vi "Get DDG External Output Time.vi"(8 "error in (no error)":errorcluster, 9 "puiWidth":cluster{}, 10 "puiDelay":cluster{}, 11 "uiIndex":u32) -> (0 "error out":errorcluster, 1 "puiWidth out":cluster{}, 2 "puiDelay out":cluster{}, 3 "function return":u32)   [LabVIEW 2014, in "atmcd32d.lvlib"]
doc: "unsigned int WINAPI GetDDGExternalOutputTime(at_u32 uiIndex, at_u64 * puiDelay, at_u64 * puiWidth);"
uses:
  atmcd32d.lvlib
  atmcd32d.dll
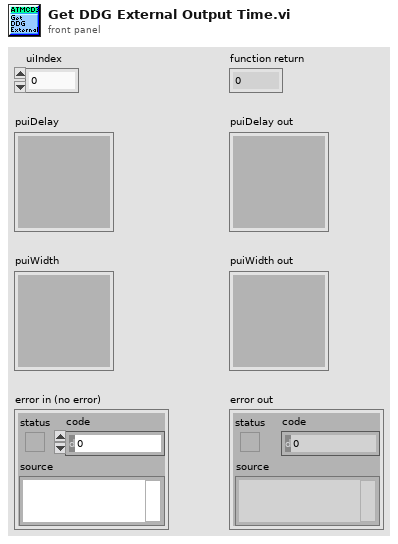
[diagram p1: front panel]
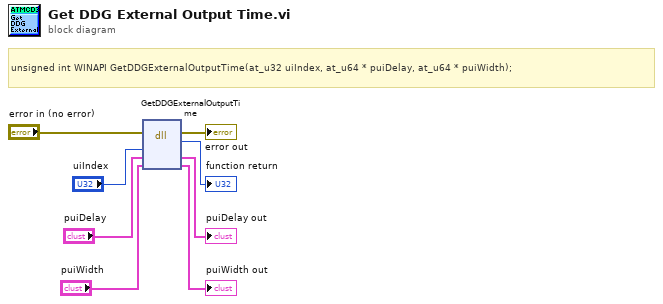
[diagram p0: block diagram]
diagram:
  # "unsigned int WINAPI GetDDGExternalOutputTime(at_u32 uiIndex, at_u64 * puiDelay, at_u64 * puiWidth);"
  n1 = dll-call lib="C:/Users/Bakir/Documents/Lambda2-Testing/lib/Andorlib/atmcd32d.*" fn="GetDDGExternalOutputTime"(error in="error in (no error)", "uiIndex"="uiIndex", "puiDelay"="puiDelay", "puiWidth"="puiWidth") -> (error out=→"error out":errorcluster, →"function return":u32, "puiDelay"=→"puiDelay out":cluster{}, "puiWidth"=→"puiWidth out":cluster{})  [unwired: 3 in, 1 out]
